vi "Insert Coin.vi"(8 "error in (no error)":errorcluster, 11 "TestCase in":refnum<class "Test DataBase.lvclass">) -> (0 "error out":errorcluster, 3 "TestCase out":refnum<class "Test DataBase.lvclass">)   [LabVIEW 2020, in "Test DataBase.lvclass"]
uses:
  Test DataBase.lvclass
  Dinero/Dinero.lvclass
  Dinero/Dinero.lvclass/Dinero.ctl
  <vilib>/addons/_JKI Toolkits/VI Tester/TestCase.llb/TestCase.lvclass
  C:/Program Files (x86)/National Instruments/LabVIEW 2020/vi.lib/addons/_JKI Toolkits/VI Tester/TestCase.llb/TestCase.lvclass
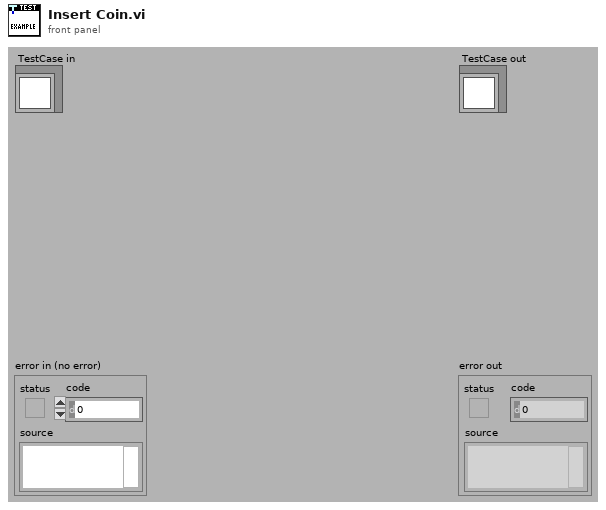
[diagram p1: front panel]
types:
  T1 = cluster{"Moneda 1":bool, "Moneda 2":bool, "Moneda 5":bool, "Moneda 10":bool, "Billete 20":bool, "Billete 50":bool, "Billete 100":bool, "Billete 200":bool}
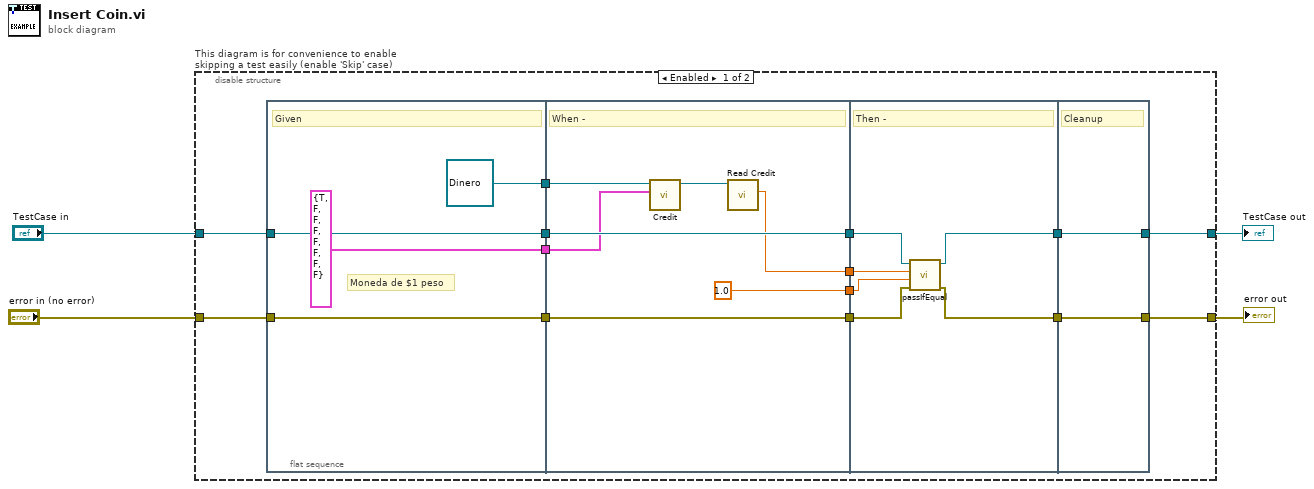
[diagram p0: block diagram]
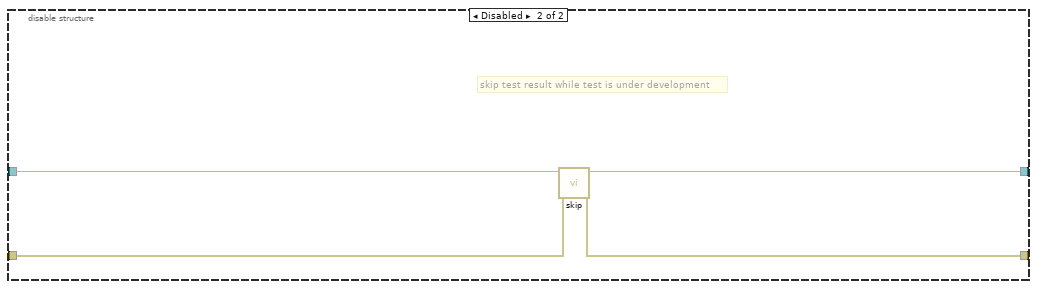
[diagram p2: hidden frame]
diagram:
  n1 = disable-structure "This diagram is for convenience to enable skipping a test easily (enable 'Skip' case)" shown="Enabled" {
    disable-tunnel: "TestCase in" -> [w12 w41]
    disable-tunnel: [w9 w39] -> w1
    disable-tunnel: [w10 w40] -> w3
    disable-tunnel: "error in (no error)" -> [w11 w38]
    frame Enabled {
      n2 = flat-sequence {
        tunnel: w11 -> [w21]
        tunnel: w12 -> [w22]
        tunnel: [w22] -> w18
        tunnel: [w21] -> w17
        tunnel: [T1 {"Moneda 1"=TRUE, "Moneda 2"=FALSE, "Moneda 5"=FALSE, "Moneda 10"=FALSE, "Billete 20"=FALSE, "Billete 50"=FALSE, "Billete 100"=FALSE, "Billete 200"=FALSE} ("Monedas")] -> w8
        tunnel: [refnum<class "Dinero.lvclass"> refnum ("Dinero.lvlib:Dinero.lvclass")] -> w5
        tunnel: [w29] -> w16
        tunnel: [w28] -> w15
        tunnel: w18 -> [w29]
        tunnel: w17 -> [w28]
        tunnel: w8 -> [w27]
        tunnel: [w25] -> w7
        tunnel: [1.0] -> w6
        tunnel: w5 -> [w23]
        tunnel: [w34] -> w14
        tunnel: [w32] -> w13
        tunnel: w16 -> [w35]
        tunnel: w15 -> [w33]
        tunnel: w7 -> [w31]
        tunnel: w6 -> [w30]
        tunnel: [w36] -> w10
        tunnel: [w37] -> w9
        tunnel: w14 -> [w37]
        tunnel: w13 -> [w36]
        frame #0 {
          # "Moneda de $1 peso"
          # "Given"
        }
        frame #1 {
          # "When -"
          n3 = call "Credit.vi"("Monedas"=w27, "Dinero in"=w23) -> ("Dinero out"=w26:refnum<class "Dinero.lvclass">)  [unwired: 8 in, 1 out]
          n4 = call "Read Credit.vi"("Dinero in"=w26) -> ("Credit"=w25:dbl)  [unwired: 8 in, 2 out]
        }
        frame #2 {
          # "Then -"
          n5 = call-dynamic "passIfEqual.vi"("error in (no error)"=w33, "y"=w30, "x"=w31, "TestCase in"=w35) -> ("error out"=w32:errorcluster, "TestCase out"=w34:refnum<class "Test DataBase.lvclass">)  [unwired: 6 in]
        }
        frame #3 {
          # "Cleanup"
        }
      }
    }
    frame Disabled {
      # "skip test result while test is under development"
      n6 = call <vilib>:"skip.vi"("error in (no error)"=w38, "TestCase in"=w41) -> ("error out"=w40:errorcluster, "TestCase out"=w39:refnum<class "Test DataBase.lvclass">)  [unwired: 8 in]
    }
  }
  "error out" <- w3
  "TestCase out" <- w1
